vi "Set Counter Signal.vi"(6 "Protections":T1, 8 "error in (no error)":errorcluster, 9 "Counter Value":dbl, 10 "Frame.Data in":dbl[](array[numeric]), 11 "Counter Configuration in":T2) -> (0 "error out":errorcluster, 2 "Frame.Data out":dbl[](array[numeric]), 3 "Counter Configuration out":T2)   [LabVIEW 2019, in "Protection and Counter Support Engine.lvlib"]
uses:
  Protection and Counter Support Engine.lvlib
  Shared/Types/Exported Counter Settings.ctl
  <vilib>/NI/NIVS Inline Async API/_Data Access Engine/Data Access Engine/Types/Write.DVR.ctl
  <vilib>/NI/NIVS Inline Async API/_Data Access Engine/Access Type Classes/Write/Write.lvclass
  <vilib>/NI/NIVS Inline Async API/_Data Access Engine/Access Type Classes/Write/Write.lvclass/Write.ctl
  <vilib>/NI/NIVS Inline Async API/_Data Access Engine/Data Access Engine/Methods/Write.Data.Buffer.vi
  <vilib>/NI/NIVS Inline Async API/_Data Access Engine/Access Type Classes/Write/Write.Buffer.vi
  <vilib>/NI/NIVS Inline Async API/_Data Access Engine/Data Access Engine/Data Access Engine.lvclass
  Shared/Protection and Counter Support Shared.lvlib
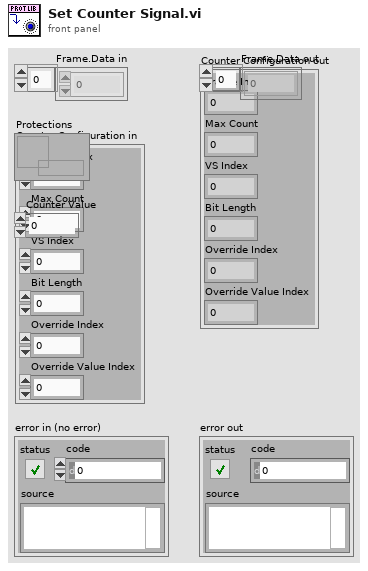
[diagram p1: front panel]
types:
  T1 = typedef "Data Access Engine.lvlib/Data Access Engine.lvclass/Write.DVR.ctl" = refnum<data-value>
  T2 = typedef "Protection and Counter Support Shared.lvlib/Exported Counter Settings.ctl" = cluster{"Frame Index":i32, "Max Count":dbl, "VS Index":i32, "Bit Length":i64, "Override Index":i32, "Override Value Index":i32}
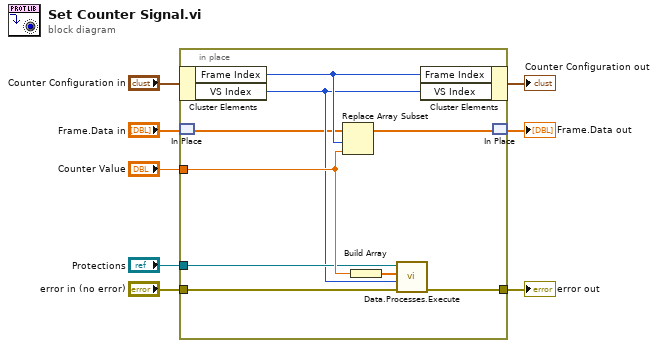
[diagram p0: block diagram]
diagram:
  n1 = in-place {
    in-place-border: "Counter Value" -> [w17]
    in-place-border: "error in (no error)" -> [w15]
    in-place-border: [w14] -> w3
    in-place-border: "Protections" -> [w13]
    n2 = in-place-cluster #1("Counter Configuration in") -> ("Frame Index"=w12:i32, "VS Index"=w11:i32)
    n3 = in-place-match #2("Frame.Data in") -> (w10:dbl[])
    n4 = Replace Array Subset(array=w10, new element=w17, index=w12) -> (w9:dbl[])
    n5 = Build Array(w17) -> (w16:dbl[])
    n6 = call-poly <vilib>:"Data.Processes.Execute.vi"("error in (no error)"=w15, "Offset"=w11, "Values"=w16, "Ref"=w13) -> ("error out"=w14:errorcluster)  [unwired: 7 in]
    n7 = in-place-cluster #1("Frame Index"=w12, "VS Index"=w11) -> (→"Counter Configuration out":T2)
    n8 = in-place-match #2(w9) -> (→"Frame.Data out":dbl[])
  }
  "error out" <- w3
